vi "Client Serialization Test.vi"() -> (0 "Validation Error":errorcluster, 1 "Init/SerDes Error":errorcluster, 2 "Test Results":T1)   [LabVIEW 2014, in "OPC UA Client Tests.lvlib"]
doc: "Test Serialization and Deserialization of Configuration class"
uses:
  OPC UA Client Tests.lvlib
  module/configuration/OPC UA Client configuration.lvclass
  module/configuration/OPC UA Client configuration.lvclass/OPC UA Client configuration.ctl
  <vilib>/NI/Tag Bus Module Framework/channel/TBM channel.lvclass
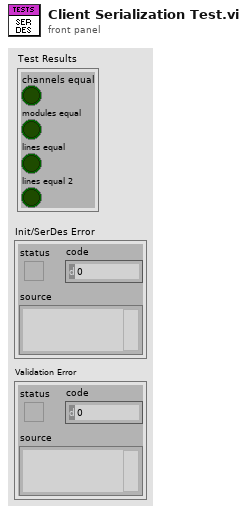
[diagram p1: front panel]
types:
  T1 = cluster{"channels equal":bool, "modules equal":bool, "lines equal":bool, "lines equal 2":bool}
  T2 = typedef "OPC UA Client configuration.lvclass/Line.ctl" = cluster{"channel":refnum<class "TBM channel.lvclass">, "Node Path":string, "OPC UA Data Type":T3}
  T3 = typedef "OPC UA Client configuration.lvclass/OPC UA Data Type.ctl" = u16
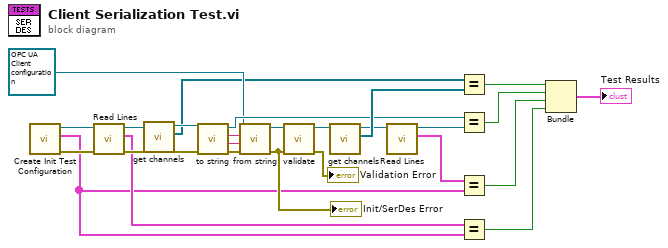
[diagram p0: block diagram]
diagram:
  n1 = call "Create Init Test Configuration.vi"() -> ("error out"=w11:errorcluster, "Lines"=w6:T2[], "module"=w9:refnum<class "OPC UA Client configuration.lvclass">)  [unwired: 9 in]
  n2 = call "Read Lines.vi"("error in (no error)"=w11, "OPC UA configuration in"=w9) -> ("error out"=w10:errorcluster, "Lines"=w7:T2[], "OPC UA configuration out"=w8:refnum<class "OPC UA Client configuration.lvclass">)  [unwired: 7 in]
  n3 = call-dynamic "get channels.vi"("OPC UA configuration in"=w8) -> ("channels"=w15:refnum<class "TBM channel.lvclass">[], "OPC UA configuration out"=w16:refnum<class "OPC UA Client configuration.lvclass">)  [unwired: 9 in]
  n4 = call-dynamic "to string.vi"("error in"=w10, "OPC UA configuration in"=w16) -> ("error out"=w26:errorcluster, "data"=w25:string, "version"=w24:string, "OPC UA configuration out"=w18:refnum<class "OPC UA Client configuration.lvclass">)  [unwired: 6 in]
  n5 = call-dynamic "from string.vi"("error in"=w26, "data"=w25, "version"=w24, "OPC UA configuration in"=refnum<class "OPC UA Client configuration.lvclass"> refnum ("tag bus configurable plugin module configuration")) -> ("error out"=w21:errorcluster, "OPC UA configuration out"=w23:refnum<class "OPC UA Client configuration.lvclass">)  [unwired: 6 in]
  "Init/SerDes Error" <- w21
  n6 = call-dynamic "validate.vi"("error in"=w21, "OPC UA configuration in"=w23) -> ("error out"=→"Validation Error":errorcluster, "OPC UA configuration out"=w20:refnum<class "OPC UA Client configuration.lvclass">)  [unwired: 8 in]
  n7 = call-dynamic "get channels.vi"("OPC UA configuration in"=w20) -> ("channels"=w19:refnum<class "TBM channel.lvclass">[], "OPC UA configuration out"=w14:refnum<class "OPC UA Client configuration.lvclass">)  [unwired: 9 in]
  n8 = call "Read Lines.vi"("OPC UA configuration in"=w14) -> ("Lines"=w12:T2[], "OPC UA configuration out"=w13:refnum<class "OPC UA Client configuration.lvclass">)  [unwired: 8 in, 1 out]
  n9 = Equal?(x=w15, y=w19) -> (x = y?=w5:bool)
  n10 = Equal?(x=w18, y=w13) -> (x = y?=w4:bool)
  n11 = Equal?(x=w12, y=w6) -> (x = y?=w3:bool)
  n12 = Equal?(x=w7, y=w6) -> (x = y?=w2:bool)
  n13 = Bundle(w5, w4, w3, w2) -> (→"Test Results":cluster{bool, bool, bool, bool})  [unwired: 1 in]
